vi "Parse Session (Tx-UDP).vi"(8 "error in":errorcluster, 11 "node in":refnum<k20>) -> (0 "error out":errorcluster, 3 "tx udp session out":T1={"VlId"=0, "Bag"=0, "NetSelect"=0, "domainID"=1, "sideID"=1, "locationID"=1, "interfaceID"=1, "NumOfSubVl"=0, "Skew"=0, "MaxFrameLength"=0, "FrameBufferSize"=0} {"NumOfSubVl" format="%.0b"; "NetSelect" items=["FDX_TX_FRAME_DLY_A", "FDX_TX_FRAME_DLY_B", "FDX_TX_FRAME_BOTH", "FDX_TX_FRAME_ONLY_A", "FDX_TX_FRAME_ONLY_B"]})   [LabVIEW 2020, in "AIM ARINC 664 Import.lvlib"]
uses:
  AIM ARINC 664 Import.lvlib
  _typedefs/tx_udp_setup.ctl
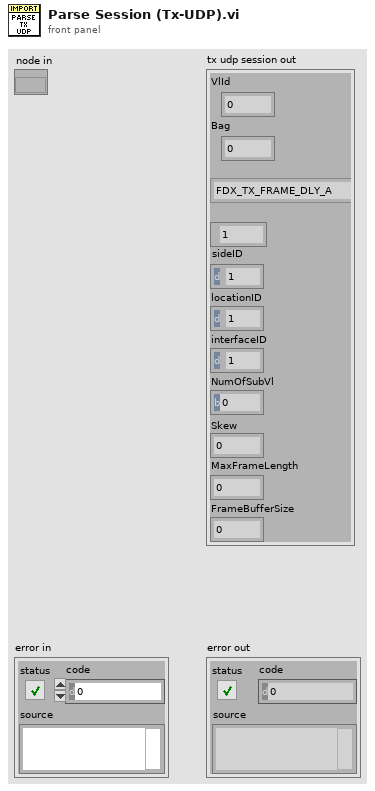
[diagram p1: front panel]
types:
  T1 = typedef "AIM ARINC 664 Import.lvlib/tx_udp_setup.ctl" = cluster{"VlId":i32, "Bag":i32, "NetSelect":u32, "domainID":u8, "sideID":u8, "locationID":u8, "interfaceID":u8, "NumOfSubVl":u16, "Skew":u32, "MaxFrameLength":u32, "FrameBufferSize":u32}
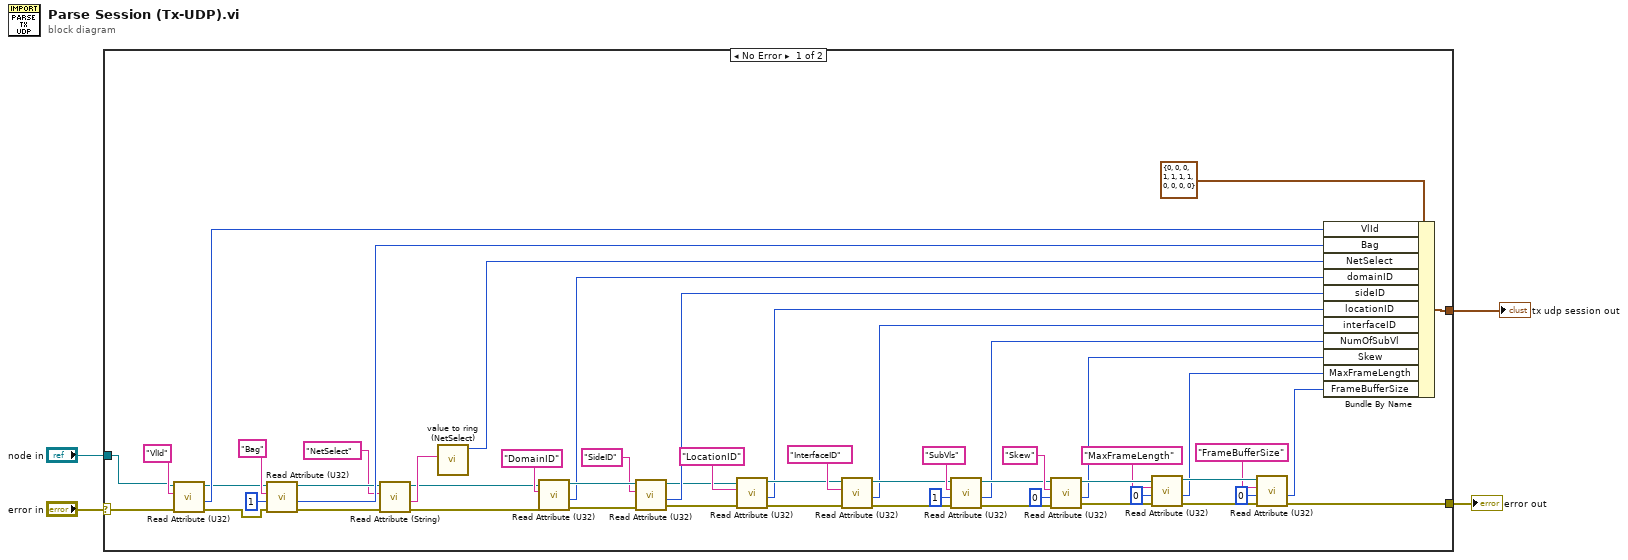
[diagram p0: block diagram]
diagram:
  n1 = case shown="No Error" "error in" {
    selector: "error in" -> [w49 w58]
    tunnel: "node in" -> [w48 _]
    tunnel: [w18 w58] -> w3
    tunnel: [w50 _] -> w1
    frame No Error {
      n2 = call "Read Attribute (U32).vi"("error in"=w49, "Attribute Name"="VlId" ("Tag Name"), "node in"=w48) -> ("error out"=w8:errorcluster, "value"=w53:u32, "node out"=w9:refnum<k20>)  [unwired: 6 in]
      n3 = call "Read Attribute (U32).vi"("error in"=w8, "default"=u32 1, "Attribute Name"="Bag" ("Tag Name"), "node in"=w9) -> ("error out"=w56:errorcluster, "value"=w57:u32, "node out"=w55:refnum<k20>)  [unwired: 5 in]
      n4 = call "Read Attribute (String).vi"("error in"=w56, "Attribute Name"="NetSelect" ("Tag Name"), "node in"=w55) -> ("error out"=w6:errorcluster, "value"=w17:string, "node out"=w7:refnum<k20>)  [unwired: 6 in]
      n5 = call "value to ring (NetSelect).vi"("value"=w17) -> ("NetSelect"=w16:u32)  [unwired: 10 in]
      n6 = call "Read Attribute (U32).vi"("error in"=w6, "Attribute Name"="DomainID" ("Tag Name"), "node in"=w7) -> ("error out"=w47:errorcluster, "value"=w44:u32, "node out"=w46:refnum<k20>)  [unwired: 6 in]
      n7 = call "Read Attribute (U32).vi"("error in"=w47, "Attribute Name"="SideID" ("Tag Name"), "node in"=w46) -> ("error out"=w37:errorcluster, "value"=w42:u32, "node out"=w38:refnum<k20>)  [unwired: 6 in]
      n8 = call "Read Attribute (U32).vi"("error in"=w37, "Attribute Name"="LocationID" ("Tag Name"), "node in"=w38) -> ("error out"=w35:errorcluster, "value"=w36:u32, "node out"=w40:refnum<k20>)  [unwired: 6 in]
      n9 = call "Read Attribute (U32).vi"("error in"=w35, "Attribute Name"="InterfaceID" ("Tag Name"), "node in"=w40) -> ("error out"=w23:errorcluster, "value"=w15:u32, "node out"=w24:refnum<k20>)  [unwired: 6 in]
      n10 = call "Read Attribute (U32).vi"("error in"=w23, "default"=u32 1, "Attribute Name"="SubVls" ("Tag Name"), "node in"=w24) -> ("error out"=w25:errorcluster, "value"=w22:u32, "node out"=w26:refnum<k20>)  [unwired: 5 in]
      n11 = call "Read Attribute (U32).vi"("error in"=w25, "default"=u32 0, "Attribute Name"="Skew" ("Tag Name"), "node in"=w26) -> ("error out"=w33:errorcluster, "value"=w21:u32, "node out"=w32:refnum<k20>)  [unwired: 5 in]
      n12 = call "Read Attribute (U32).vi"("error in"=w33, "default"=u32 0, "Attribute Name"="MaxFrameLength" ("Tag Name"), "node in"=w32) -> ("error out"=w34:errorcluster, "value"=w20:u32, "node out"=w30:refnum<k20>)  [unwired: 5 in]
      n13 = call "Read Attribute (U32).vi"("error in"=w34, "default"=u32 0, "Attribute Name"="FrameBufferSize" ("Tag Name"), "node in"=w30) -> ("error out"=w18:errorcluster, "value"=w19:u32)  [unwired: 5 in, 1 out]
      n14 = Bundle By Name(cluster=T1 {"VlId"=0, "Bag"=0, "NetSelect"=0, "domainID"=1, "sideID"=1, "locationID"=1, "interfaceID"=1, "NumOfSubVl"=0, "Skew"=0, "MaxFrameLength"=0, "FrameBufferSize"=0} ("tx_udp_setup"), "VlId"=w53, "Bag"=w57, "NetSelect"=w16, "domainID"=w44, "sideID"=w42, "locationID"=w36, "interfaceID"=w15, "NumOfSubVl"=w22, "Skew"=w21, "MaxFrameLength"=w20, "FrameBufferSize"=w19) -> (w50:T1)
    }
    frame Error {
    }
  }
  "error out" <- w3
  "tx udp session out" <- w1
